vi "ReadSalicruAPI (SubVI).vi"(8 "error in (no error)":errorcluster, 10 "Python File":path, 11 "session in":refnum<k35>) -> (0 "error out":errorcluster, 1 "Array":i32[](array[numeric]), 2 "Map":map{string, dbl}(c390), 3 "session out":refnum<k35>)   [LabVIEW 2024, in "SALICRUAPI.lvlib"]
uses:
  SALICRUAPI.lvlib
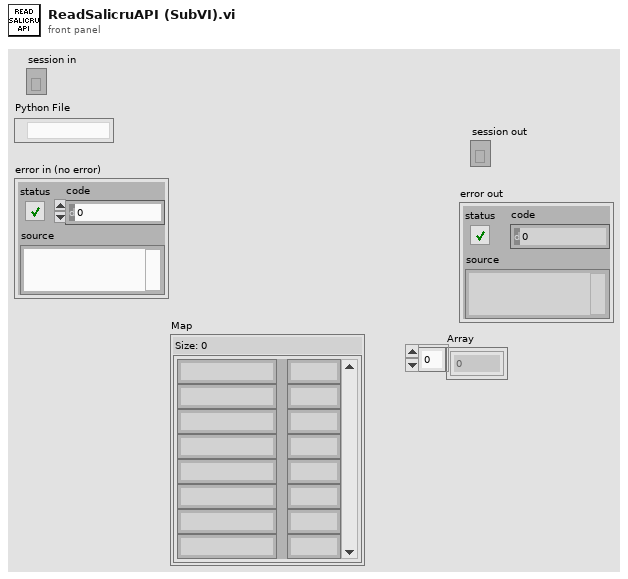
[diagram p1: front panel]
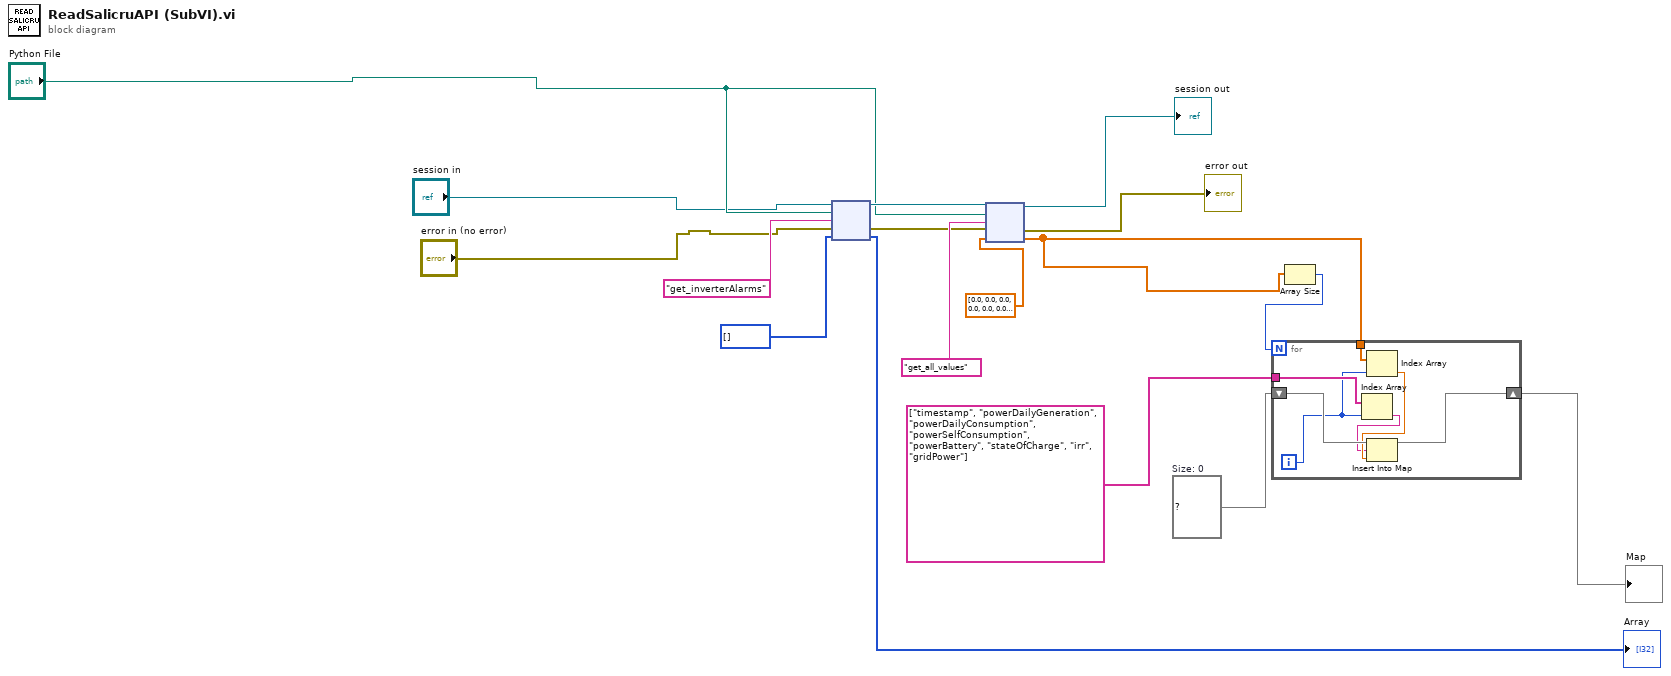
[diagram p0: block diagram]
diagram:
  w14 = map{string, dbl} {}  # Size: 0
  n1 = node("session in", "Python File", "get_inverterAlarms" ("function name"), "error in (no error)", i32[] []) -> (w7:refnum<k35>, w8:errorcluster, →"Array":i32[])  [unwired: 2 out]
  n2 = node(w7, "Python File", "get_all_values" ("function name"), w8, dbl[] [0.0, 0.0, 0.0, 0.0, 0.0, 0.0, 0.0, 0.0]) -> (→"session out":refnum<k35>, →"error out":errorcluster, w15:dbl[])  [unwired: 2 out]
  n3 = Array Size(array=w15) -> (size(s)=w13:i32)
  n4 = for {
    N: w13 -> [_]
    shift-right: [w24] -> w17
    shift-left: w14 -> [w23]
    tunnel: w15 -> [w22]
    tunnel: string[] ["timestamp", "powerDailyGeneration", "powerDailyConsumption", "powerSelfConsumption", "powerBattery", "stateOfCharge", "irr", "gridPower"] -> [w21]
    i -> [w20]
    n5 = Index Array(array=w21, index=w20) -> (element=w18:string)
    n6 = Index Array(array=w22, index=w20) -> (element=w19:dbl)
    n7 = Insert Into Map(map in=w23, key=w18, value=w19) -> (map out=w24:map{string, dbl})  [unwired: 2 out]
  }
  "Map" <- w17
